vi "N330X_Enable_Disable.vi"(8 "error in (no error) 2":errorcluster, 9 "Enable Input (Enable)":bool=TRUE, 10 "Channel (1)":u32=1, 11 "VISA resource name 2":refnum<visa-resource-name>) -> (0 "error out":errorcluster)   [LabVIEW 2015]
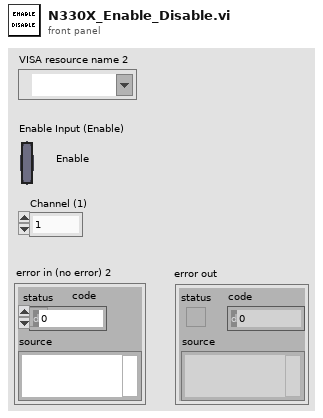
[diagram p1: front panel]
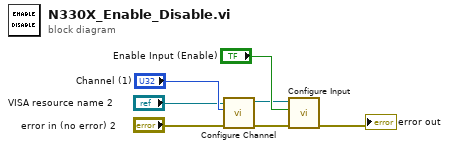
[diagram p0: block diagram]
diagram:
  n1 = call <instrlib>:"Configure Channel.vi"("error in (no error)"="error in (no error) 2", "Channel (1)"="Channel (1)", "VISA resource name"="VISA resource name 2") -> ("error out"=w1:errorcluster, "VISA resource name out"=w2:refnum<visa-resource-name>)  [unwired: 7 in]
  n2 = call <instrlib>:"Configure Input.vi"("error in (no error)"=w1, "Enable Input (Enable)"="Enable Input (Enable)", "VISA resource name"=w2) -> ("error out"=→"error out":errorcluster)  [unwired: 7 in, 1 out]
